vi "dfd_Get Filter Freq Resp on Freq Pts from TF.vi"(6 "fs [Hz]":dbl=1.0 format="%.2f", 7 "factor":i32, 8 "error in (no error)":errorcluster, 9 "den":dbl[](array[numeric])=[1.0] format="%.2f", 10 "num":dbl[](array[numeric]) format="%.2f", 11 "freq points [Hz]":dbl[](array[numeric]) format="%.2f") -> (0 "error out":errorcluster, 3 "freq response":cdb[](array[numeric]) format="%.2f")   [LabVIEW 2017, in "NI_DigFilterLicensed.lvlib"]
uses:
  <vilib>/addons/Digital Filter Design/NI_DigFilterLicensed.lvlib
  <vilib>/Analysis/1siggen.llb/Ramp Pattern by Samples.vi
  <vilib>/Analysis/NI_AALBase.lvlib
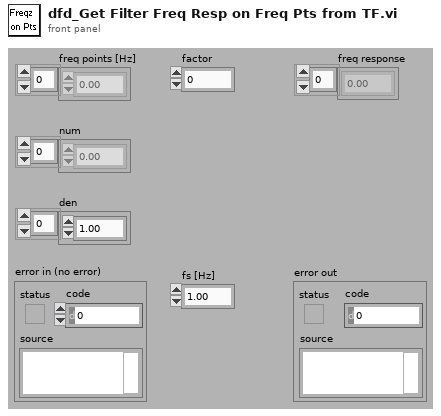
[diagram p1: front panel]
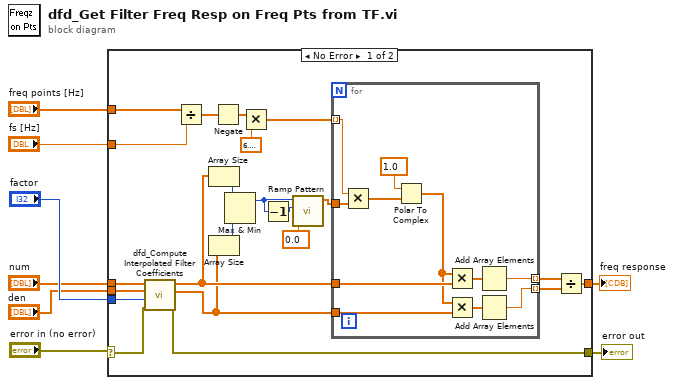
[diagram p0: block diagram]
diagram:
  n1 = case shown="No Error" "error in (no error)" {
    selector: "error in (no error)" -> [w10 w42]
    tunnel: [w19 _] -> w8
    tunnel: "fs [Hz]" -> [w17 _]
    tunnel: "freq points [Hz]" -> [w16 _]
    tunnel: "factor" -> [w13 _]
    tunnel: "num" -> [w12 _]
    tunnel: "den" -> [w11 _]
    tunnel: [w9 w42] -> w1
    frame No Error {
      n2 = call <vilib>:"dfd_Compute Interpolated Filter Coefficients.vi"("error in (no error)"=w10, "factor"=w13, "denominator in"=w11, "numerator in"=w12) -> ("error out"=w9:errorcluster, "denominator out"=w14:dbl[], "numerator out"=w15:dbl[])  [unwired: 5 out]
      n3 = Divide(x=w16, y=w17) -> (x/y=w18:dbl[])
      n4 = Array Size(array=w15) -> (size(s)=w27:i32)
      n5 = Array Size(array=w14) -> (size(s)=w26:i32)
      n6 = Negate(x=w18) -> (-x=w20:dbl[])
      n7 = Max & Min(x=w27, y=w26) -> (max(x,y)=w28:i32)  [unwired: 1 out]
      n8 = Multiply(x=w20, y=6.283185307179586) -> (x*y=w23:dbl[])
      n9 = Decrement(x=w28) -> (x-1=w22:i32)
      n10 = call-poly <vilib>:"Ramp Pattern.vi"("start"=0.0, "end"=w22, "samples"=w28) -> ("Ramp Pattern"=w24:dbl[])  [unwired: 7 in, 1 out]
      n11 = for {
        tunnel: w23 -> [w41] mode=indexing
        tunnel: w24 -> [w40]
        tunnel: w15 -> [w38]
        tunnel: w14 -> [w39]
        tunnel: [w33] -> w29 mode=indexing
        tunnel: [w32] -> w30 mode=indexing
        n12 = Multiply(x=w41, y=w40) -> (x*y=w34:dbl[])
        n13 = Polar To Complex(1:w34, 2:1.0) -> (0:w31:cdb[])
        n14 = Multiply(x=w31, y=w38) -> (x*y=w37:cdb[])
        n15 = Multiply(x=w31, y=w39) -> (x*y=w36:cdb[])
        n16 = Add Array Elements(numeric array=w37) -> (sum=w33:cdb)
        n17 = Add Array Elements(numeric array=w36) -> (sum=w32:cdb)
      }
      n18 = Divide(x=w29, y=w30) -> (x/y=w19:cdb[])
    }
    frame Error {
    }
  }
  "freq response" <- w8
  "error out" <- w1
